vi "Build Waveform Array.vi"() -> ()   [LabVIEW 2014]
panel:
  in  "Type code Array":i32[](array[numeric])
  in  "Period":i64
  in  "current time":timestamp
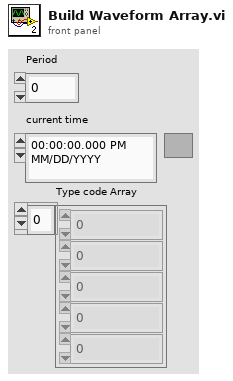
[diagram p1: front panel]
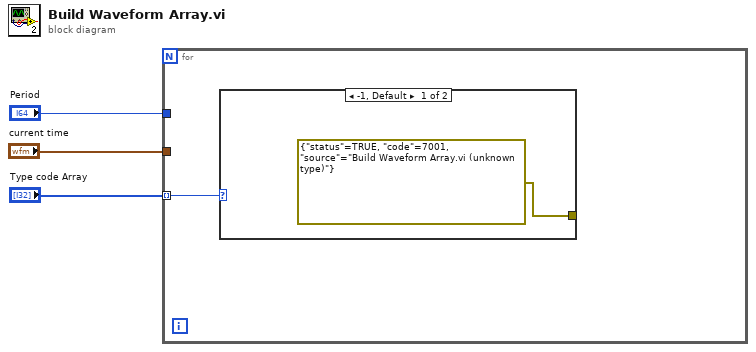
[diagram p0: block diagram]
diagram:
  n1 = for {
    tunnel: "Period" -> [_]
    tunnel: "current time" -> [_]
    tunnel: "Type code Array" -> [w4] mode=indexing
    n2 = case shown="-1, Default" w4 {
      tunnel: [errorcluster {"status"=TRUE, "code"=7001, "source"="Build Waveform Array.vi (unknown type)"} ("error constant") _] -> _
      frame -1, Default {
      }
      frame 1 {
      }
    }
  }
